vi "RESETALL.vi"(8 "error in (no error)":errorcluster, 10 "RESETALL":bool, 11 "Operation":T1) -> (0 "error out":errorcluster, 3 "RESETALL?":bool=TRUE)   [LabVIEW 2019]
uses:
  Global Operations.ctl
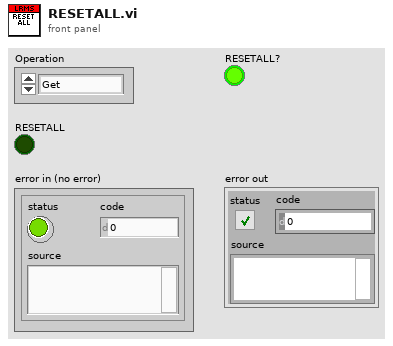
[diagram p1: front panel]
types:
  T1 = typedef "Global Operations.ctl" = enum16{"Get", "Set"}
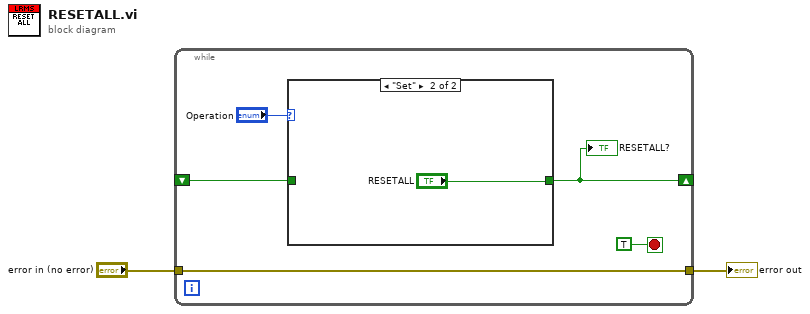
[diagram p0: block diagram]
diagram:
  n1 = while {
    shift-right: [w5] -> _
    shift-left: _ -> [w4]
    tunnel: "error in (no error)" -> [w3]
    tunnel: [w3] -> w2
    stop <- TRUE stop-if-true
    n2 = case shown="\"Set\"" "Operation" {
      tunnel: [w8 "RESETALL"] -> w5
      tunnel: w4 -> [w8 _]
      frame "Get", Default {
      }
      frame "Set" {
      }
    }
    "RESETALL?" <- w5
  }
  "error out" <- w2
